vi "Parse State Queue.vi"(0 "State Queue":string, 1 "Timeout":i32=-1, 2 "Check Events rate":i32=-1, 7 "Error In (no error)":errorcluster) -> (3 "Timeout out":i32=-1, 4 "Remaining States":string, 6 "Current State":string, 8 "Arguments":string)   [LabVIEW 2013]
doc: "Parses the JKI State Machine state queue and returns the current state that will execute next with the associated arguments.\n\nFor instructions on how to use the JKI State Machine, examples and video tutorials, visit:\nhttp://jkisoft.com/state-machine/\n\n<B>Inputs:</B>\n <B>State Queue:</B> The entire state queue is wired to this input. This should come from the main JKI State Machine shift register.\n <B>Error In</B> The error cluster from the JKI State Machine is wired to this input. If an error occures and appears on this input, the current state output returns the \"Error Handler\" state.\n\n<B>Outputs:</B>\n <B>Remaining States:</B> Returns all the next states that should execute after the current state completes. These should be passed through the current state in the state machine. These can also be modified or augmented within the current state if necessary.\n <B>Current State:</B> Returns the current state that should execute next in the state machine. If an error is wired to the Error input then the current state output becomes \"Error Handler\".\n <B>Arguments:</B> Returns any argument(s) that may be used in the current state string. These arguments come after the \">>\" characters. <B>Note:</B> The arguments variable must not contain any unprintable characters like linefeed or carriage return.\n\n<B>State Syntax:</B>\nStateCategory: State >> Argument\nLine Terminator: Line feed\n <B>Example:</B>\nUI: Help >> About\n\nWhere \"UI\" is the state category\nWhere \"Help\" is the state\nWhere \"About\" is the argument\n <B>Other Examples:</B>\nApp Data: Initialize\nUI: Initialize\nHelp >> About\n\n<B>Commenting:</B>\nTo add a comment use \"//\" or \"#\" and all text to the right will be ignored\n <B>Commenting Example:</B>\nUI: Initialize // This initializes the UI\n# This whole line is a comment\n// Another comment line"
panel:
  # "For instructions on how to use the JKI State Machine, examples and video tutorials, visit:\nhttp://jki.net/state-machine/\n\nJKI State Machine™\nhttp://jki.net/state-machine/\nCopyright (C) 2005-2020, JKI <info@jki.net>\nALL RIGHTS RESERVED"
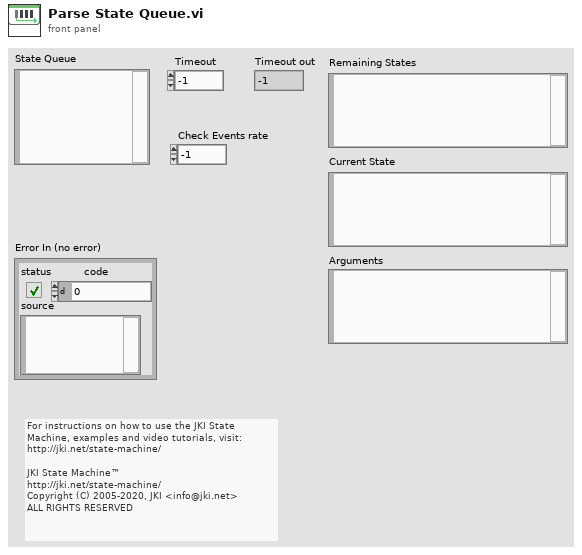
[diagram p1: front panel]
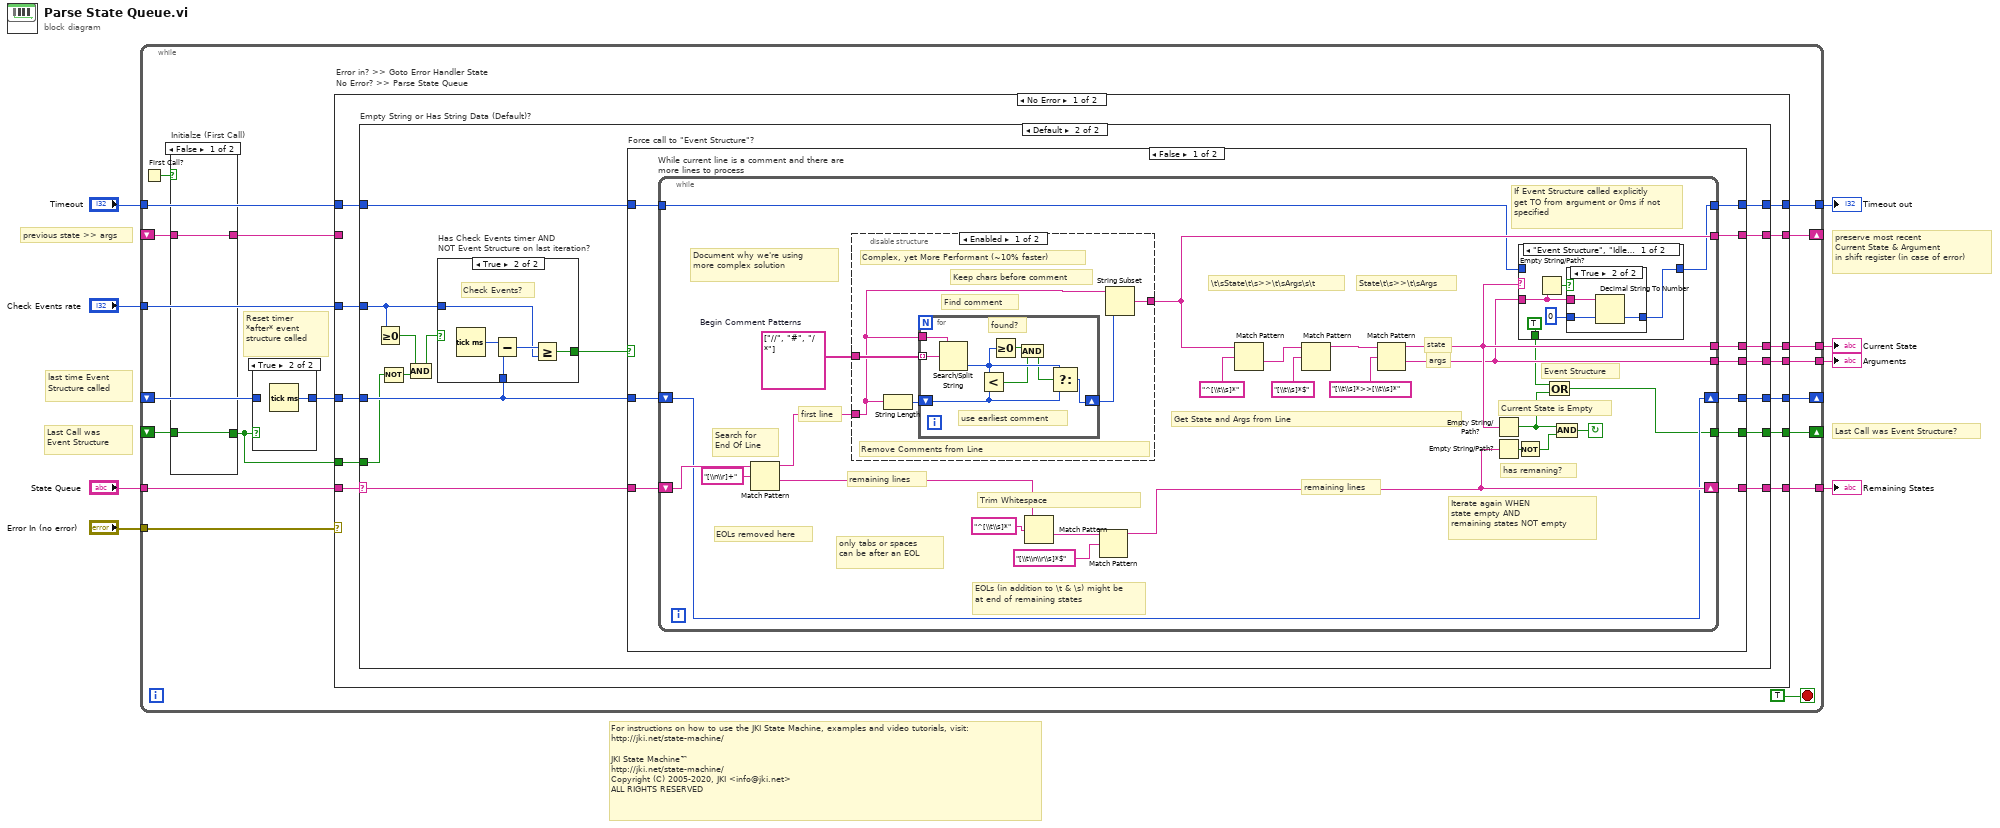
[diagram p0: block diagram]
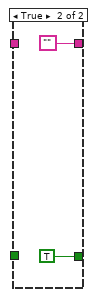
[diagram p2: hidden frame]
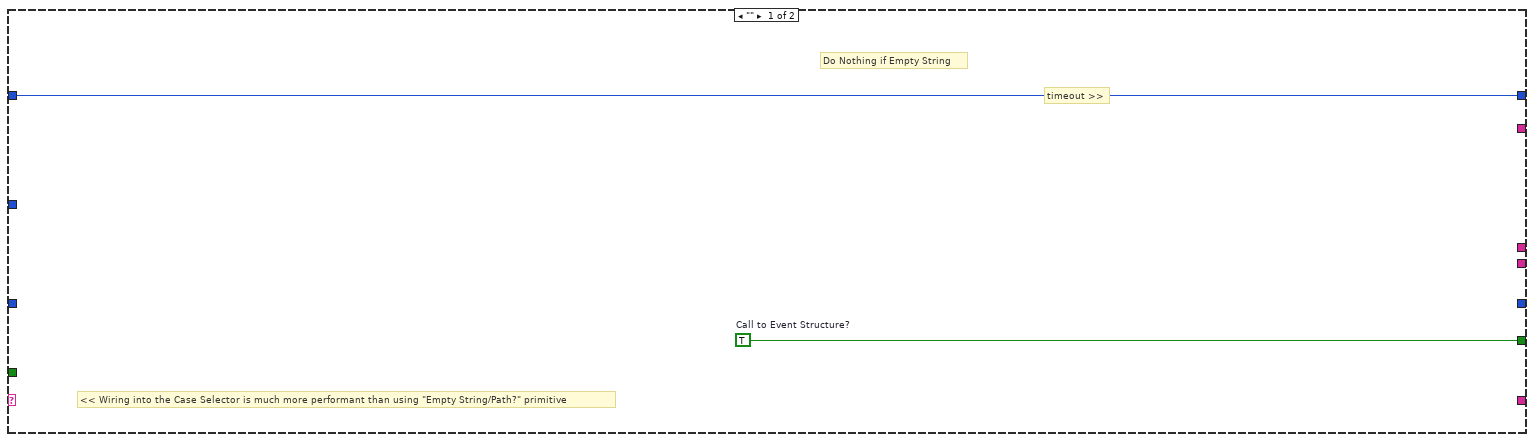
[diagram p4: hidden frame]
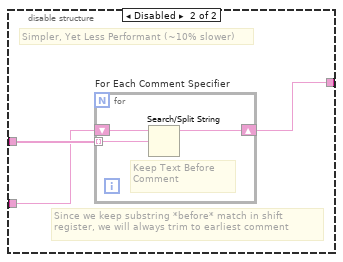
[diagram p8: hidden frame]
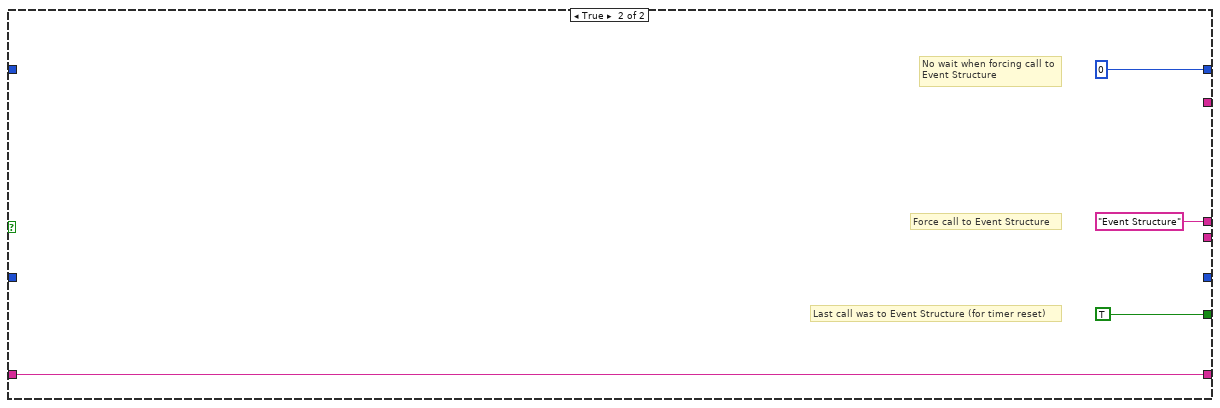
[diagram p9: hidden frame]
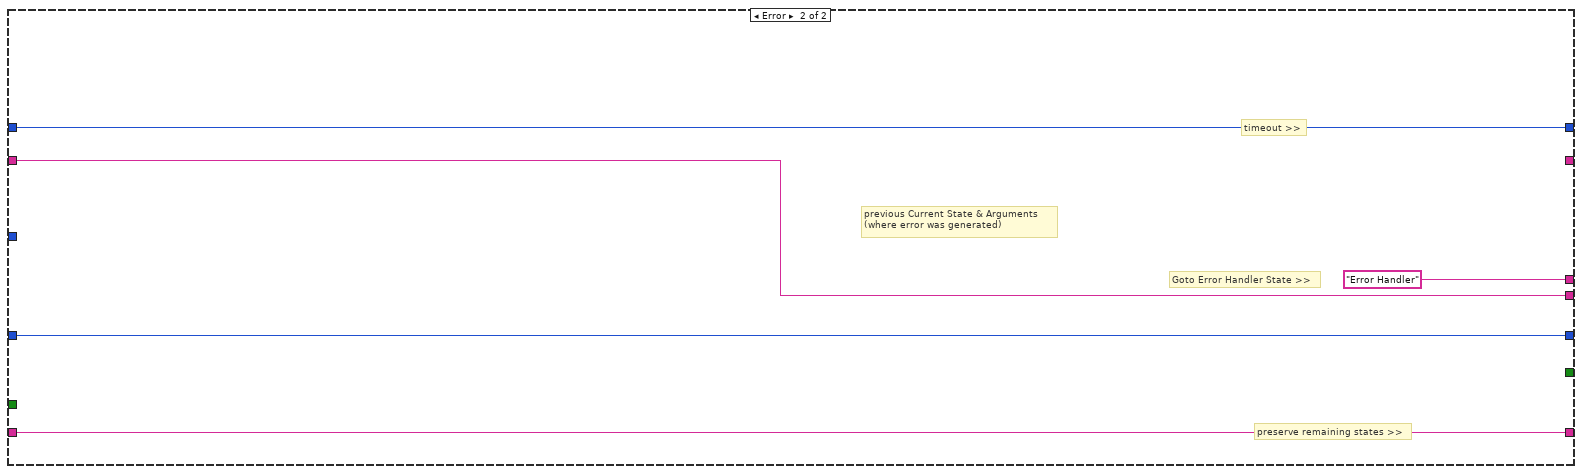
[diagram p10: hidden frame]
diagram:
  # "Last Call was Event Structure"
  # "Last Call was Event Structure?"
  # "last time Event Structure called"
  # "previous state >> args"
  # "preserve most recent\nCurrent State & Argument\nin shift register (in case of error)"
  # "For instructions on how to use the JKI State Machine, examples and video tutorials, visit:\nhttp://jki.net/state-machine/\n\nJKI State Machine™\nhttp://jki.net/state-machine/\nCopyright (C) 2005-2020, JKI <info@jki.net>\nALL RIGHTS RESERVED"
  n1 = while {
    tunnel: [w27] -> w8
    tunnel: "Error In (no error)" -> [w26]
    tunnel: "State Queue" -> [w24]
    shift-right: [w22] -> _
    shift-left: _ -> [w11]
    tunnel: [w25] -> w6
    tunnel: [w21] -> w4
    tunnel: "Timeout" -> [w20]
    tunnel: [w19] -> w2
    shift-right: [w18] -> _
    shift-left: _ -> [w14]
    tunnel: "Check Events rate" -> [w17]
    shift-right: [w16] -> _
    shift-left: _ -> [w10]
    stop <- TRUE stop-if-true
    # "Reset timer *after* event structure called"
    n2 = First Call?() -> (First Call?: T/F=w13:bool)
    n3 = case "Initialze (First Call)" shown="False" w13 {
      tunnel: [w29 ""] -> w12
      tunnel: [w28 TRUE ("f")] -> w9
      tunnel: w11 -> [w29 _]
      tunnel: w10 -> [w28 _]
      frame False {
      }
      frame True {
      }
    }
    n4 = case shown="True" w9 {
      tunnel: [w32 w33] -> w15
      tunnel: w14 -> [w32 _]
      frame False {
      }
      frame True {
        n5 = Tick Count (ms)() -> (millisecond timer value=w33:u32)
      }
    }
    n6 = case "Error in? >> Goto Error Handler State\nNo Error? >> Parse State Queue" shown="No Error" w26 {
      tunnel: [w43 w142] -> w27
      tunnel: [w45 "Error Handler"] -> w25
      tunnel: [w44 w140] -> w21
      tunnel: w24 -> [w42 w142]
      tunnel: [w41 _] -> w22
      tunnel: w12 -> [_ w140]
      tunnel: w20 -> [w40 w139]
      tunnel: [w39 w139] -> w19
      tunnel: w15 -> [w38 w138]
      tunnel: [w37 w138] -> w18
      tunnel: w17 -> [w36 _]
      tunnel: [w35 _] -> w16
      tunnel: w9 -> [w34 _]
      frame No Error {
        n7 = case "Empty String or Has String Data (Default)?" shown="Default" w42 {
          selector: w42 -> [_ w60]
          tunnel: [_ w63] -> w45
          tunnel: [_ w62] -> w44
          tunnel: [_ w61] -> w43
          tunnel: [_ w59] -> w41
          tunnel: w40 -> [w47 w58]
          tunnel: [w47 w57] -> w39
          tunnel: w38 -> [_ w54]
          tunnel: [_ w56] -> w37
          tunnel: w36 -> [_ w52]
          tunnel: [w46 w55] -> w35
          tunnel: w34 -> [_ w51]
          frame "" {
            w46 = TRUE  # Call to Event Structure?
            # "timeout >>"
            # "Do Nothing if Empty String"
            # "<< Wiring into the Case Selector is much more performant than using \"Empty String/Path?\" primitive"
          }
          frame Default {
            n8 = Greater Or Equal To 0?(x=w52) -> (x >= 0?=w49:bool)
            n9 = Not(x=w51) -> (.not. x?=w50:bool)
            n10 = Compound Arithmetic op=AND(w49, w50) -> (w48:bool)
            n11 = case "Has Check Events timer AND\nNOT Event Structure on last iteration?" shown="True" w48 {
              tunnel: [_ w66] -> w53
              tunnel: w52 -> [_ w65]
              tunnel: w54 -> [_ w64]
              frame False {
              }
              frame True {
                # "Check Events?"
                n12 = Tick Count (ms)() -> (millisecond timer value=w67:u32)
                n13 = Subtract(x=w67, y=w64) -> (x-y=w68:u32)
                n14 = Greater Or Equal?(x=w68, y=w65) -> (x >= y?=w66:bool)
              }
            }
            n15 = case "Force call to \"Event Structure\"?" shown="False" w53 {
              tunnel: [w78 "Event Structure"] -> w63
              tunnel: [w77 _] -> w62
              tunnel: [w76 w136] -> w61
              tunnel: w60 -> [w75 w136]
              tunnel: [w74 _] -> w59
              tunnel: w58 -> [w73 _]
              tunnel: [w72 0 ("Timeout")] -> w57
              tunnel: [w71 _] -> w56
              tunnel: w54 -> [w70 _]
              tunnel: [w69 TRUE] -> w55
              frame False {
                n16 = while "While current line is a comment and there are more lines to process" {
                  tunnel: [w86] -> w78
                  tunnel: [w85] -> w77
                  shift-right: [w102] -> w76
                  shift-left: w75 -> [w100]
                  tunnel: [w87] -> w74
                  tunnel: w73 -> [w83]
                  tunnel: [w84] -> w72
                  shift-right: [w80] -> w71
                  shift-left: w70 -> [w80]
                  tunnel: [w79] -> w69
                  stop <- w103 continue-if-true
                  w99 = string[] ["//", "#", "/*"]  # Begin Comment Patterns
                  # "Event Structure"
                  # "If Event Structure called explicitly get TO from argument or 0ms if not specified"
                  # "Get State and Args from Line"
                  # "State\\t\\s>>\\t\\sArgs"
                  # "\\t\\sState\\t\\s>>\\t\\sArgs\\s\\t"
                  # "remaining lines"
                  # "EOLs (in addition to \\t & \\s) might be at end of remaining states"
                  # "Document why we're using more complex solution"
                  # "Trim Whitespace"
                  # "EOLs removed here"
                  # "only tabs or spaces can be after an EOL"
                  # "Current State is Empty"
                  # "has remaning?"
                  # "remaining lines"
                  # "first line"
                  # "Search for End Of Line"
                  # "Iterate again WHEN\nstate empty AND\nremaining states NOT empty"
                  # "args"
                  # "state"
                  n17 = Match Pattern(string=w100, regular expression="[\\n\\r]+") -> (before substring=w98:string, after substring=w90:string)  [unwired: 1 in, 2 out]
                  n18 = disable-structure shown="Enabled" {
                    disable-tunnel: w99 -> [w119 w130]
                    disable-tunnel: [w118 w129] -> w87
                    disable-tunnel: w98 -> [w117 w128]
                    frame Enabled {
                      # "Remove Comments from Line"
                      # "Complex, yet More Performant (~10% faster)"
                      # "Keep chars before comment"
                      # "Find comment"
                      n19 = String Length(string=w117) -> (length=w116:i32)
                      n20 = for {
                        tunnel: w119 -> [w124] mode=indexing
                        shift-right: [w126] -> w115
                        shift-left: w116 -> [w127]
                        tunnel: w117 -> [w125]
                        # "found?"
                        # "use earliest comment"
                        n21 = Search/Split String(string=w125, search string/char (-)=w124) -> (offset of match=w123:i32)  [unwired: 1 in, 2 out]
                        n22 = Less?(x=w123, y=w127) -> (x < y?=w121:bool)
                        n23 = Greater Or Equal To 0?(x=w123) -> (x >= 0?=w122:bool)
                        n24 = And(x=w122, y=w121) -> (x .and. y?=w120:bool)
                        n25 = Select(t=w123, s=w120, f=w127) -> (s? t:f=w126:i32)
                      }
                      n26 = String Subset(string=w117, length (rest)=w115) -> (substring=w118:string)  [unwired: 1 in]
                    }
                    frame Disabled {
                      # "Since we keep substring *before* match in shift register, we will always trim to earliest comment"
                      # "Simpler, Yet Less Performant (~10% slower)"
                      n27 = for "For Each Comment Specifier" {
                        tunnel: w130 -> [w132] mode=indexing
                        shift-right: [w131] -> w129
                        shift-left: w128 -> [w133]
                        # "Keep Text Before Comment"
                        n28 = Search/Split String(string=w133, search string/char (-)=w132) -> (substring before match=w131:string)  [unwired: 1 in, 2 out]
                      }
                    }
                  }
                  n29 = Match Pattern(string=w90, regular expression="^[\\t\\s]*") -> (after substring=w89:string)  [unwired: 1 in, 3 out]
                  n30 = Match Pattern(string=w89, regular expression="[\\t\\n\\r\\s]*$") -> (before substring=w102:string)  [unwired: 1 in, 3 out]
                  n31 = Match Pattern(string=w87, regular expression="^[\\t\\s]*") -> (after substring=w88:string)  [unwired: 1 in, 3 out]
                  n32 = Match Pattern(string=w88, regular expression="[\\t\\s]*$") -> (before substring=w93:string)  [unwired: 1 in, 3 out]
                  n33 = Match Pattern(string=w93, regular expression="[\\t\\s]*>>[\\t\\s]*") -> (before substring=w86:string, after substring=w85:string)  [unwired: 1 in, 2 out]
                  n34 = Empty String/Path?(string/path=w86) -> (empty?=w81:bool)
                  n35 = Empty String/Path?(string/path=w102) -> (empty?=w104:bool)
                  n36 = Not(x=w104) -> (.not. x?=w97:bool)
                  n37 = case shown="\"Event Structure\", \"Idle\"" w86 {
                    tunnel: w85 -> [w108 _]
                    tunnel: [w109 w114] -> w84
                    tunnel: w83 -> [_ w114]
                    tunnel: [TRUE _] -> w82
                    frame "Event Structure", "Idle" {
                      n38 = Empty String/Path?(string/path=w108) -> (empty?=w107:bool)
                      n39 = case shown="True" w107 {
                        tunnel: [w110 w113] -> w109
                        tunnel: w108 -> [_ w112]
                        tunnel: 0 ("default (0 I32)") -> [w110 w111]
                        frame False {
                        }
                        frame True {
                          n40 = Decimal String To Number(string=w112, default (0L)=w111) -> (number=w113:i32)  [unwired: 1 in, 1 out]
                        }
                      }
                    }
                    frame Default {
                    }
                  }
                  n41 = Or(x=w82, y=w81) -> (x .or. y?=w79:bool)
                  n42 = And(x=w81, y=w97) -> (x .and. y?=w103:bool)
                }
              }
              frame True {
                # "Last call was to Event Structure (for timer reset)"
                # "Force call to Event Structure"
                # "No wait when forcing call to Event Structure"
              }
            }
          }
        }
      }
      frame Error {
        # "timeout >>"
        # "previous Current State & Arguments\n(where error was generated)"
        # "Goto Error Handler State >>"
        # "preserve remaining states >>"
      }
    }
  }
  "Remaining States" <- w8
  "Arguments" <- w4
  "Current State" <- w6
  "Timeout out" <- w2
